vi "Color detect test.vi"(0 "Image 3":T2(plugin-control)) -> (1 "Image":T2(plugin-control), 2 "Enum":enum16{"Z", "I", "O", "S", "L", "J", "T", "N"}(ring))   [LabVIEW 2015]
uses:
  <vilib>/vision/Image Controls.llb/IMAQ Image.ctl
  <vilib>/vision/NI_Vision_Development_Module.lvlib
panel:
  in  "output cluster 2":T1(array[cluster])
  out "Area":dbl[](array[numeric])
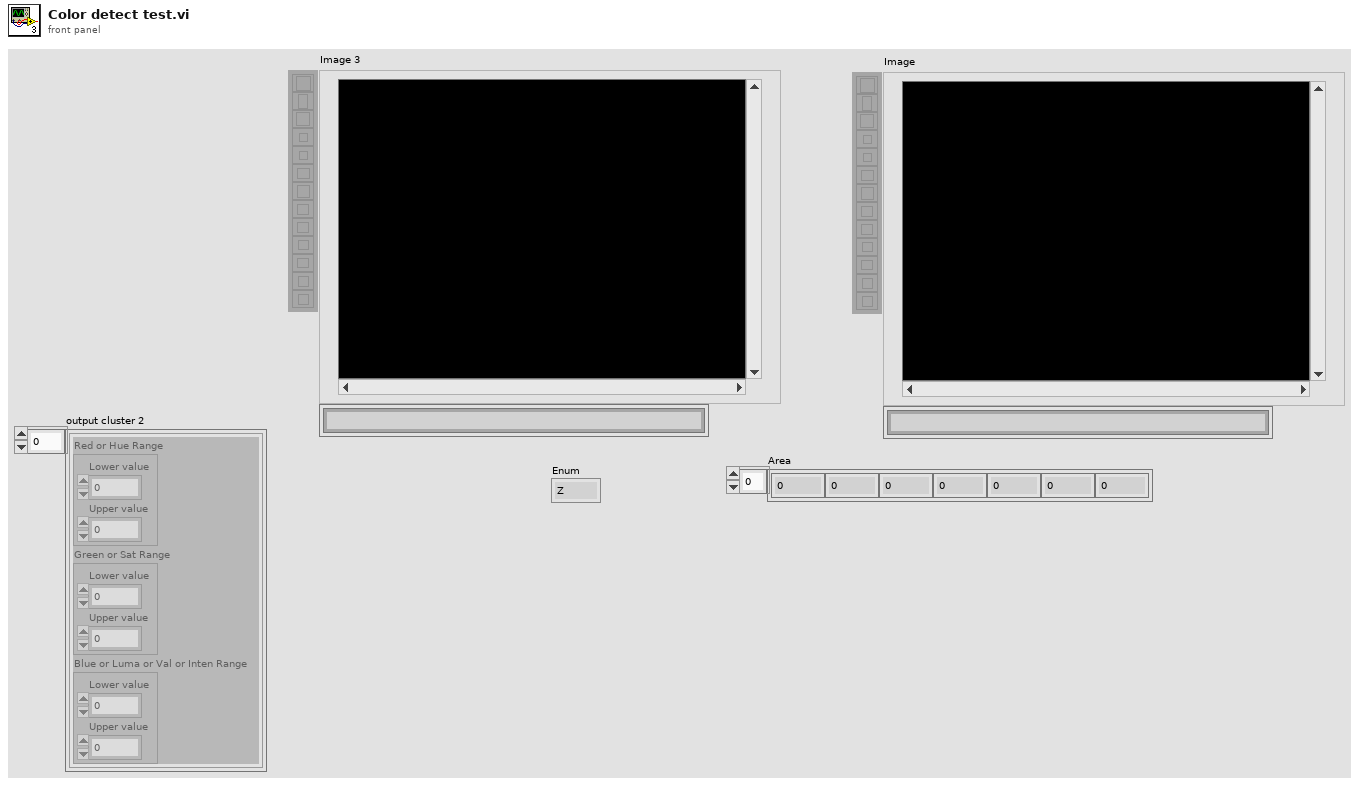
[diagram p1: front panel]
types:
  T1 = cluster{"Red or Hue Range":cluster{"Lower value":i32, "Upper value":i32}, "Green or Sat Range":cluster{"Lower value":i32, "Upper value":i32}, "Blue or Luma or Val or Inten Range":cluster{"Lower value":i32, "Upper value":i32}}[]
  T2 = typedef "IMAQ Image.ctl" = refnum<image>
  T3 = typedef "Particle Parameters" = i32
  T4 = cluster{"Red or Hue Range":cluster{"Lower value":i32, "Upper value":i32}, "Green or Sat Range":cluster{"Lower value":i32, "Upper value":i32}, "Blue or Luma or Val or Inten Range":cluster{"Lower value":i32, "Upper value":i32}}
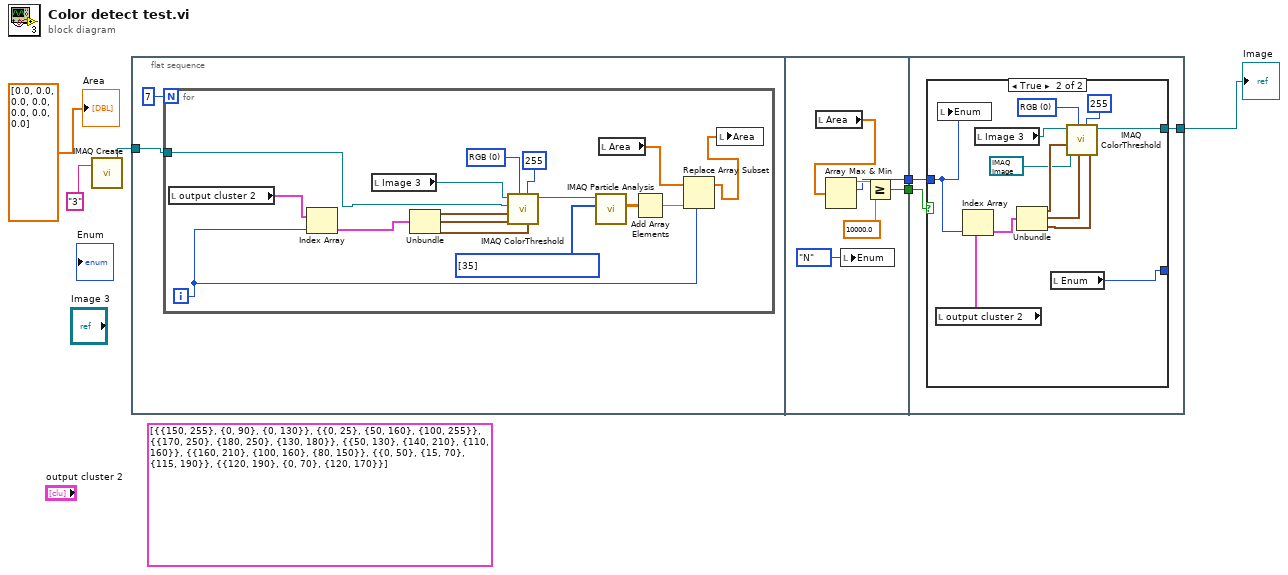
[diagram p0: block diagram]
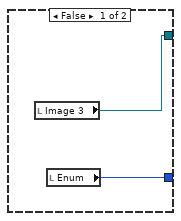
[diagram p2: hidden frame]
diagram:
  (unwired) T1 [{"Red or Hue Range"={"Lower value"=150, "Upper value"=255}, "Green or Sat Range"={"Lower value"=0, "Upper value"=90}, "Blue or Luma or Val or Inten Range"={"Lower value"=0, "Upper value"=130}}, {"Red or Hue Range"={"Lower value"=0, "Upper value"=25}, "Green or Sat Range"={"Lower value"=50, "Upper value"=160}, "Blue or Luma or Val or Inten Range"={"Lower value"=100, "Upper value"=255}}, {"Red or Hue Range"={"Lower value"=170, "Upper value"=250}, "Green or Sat Range"={"Lower value"=180, "Upper value"=250}, "Blue or Luma or Val or Inten Range"={"Lower value"=130, "Upper value"=180}}, {"Red or Hue Range"={"Lower value"=50, "Upper value"=130}, "Green or Sat Range"={"Lower value"=140, "Upper value"=210}, "Blue or Luma or Val or Inten Range"={"Lower value"=110, "Upper value"=160}}, {"Red or Hue Range"={"Lower value"=160, "Upper value"=210}, "Green or Sat Range"={"Lower value"=100, "Upper value"=160}, "Blue or Luma or Val or Inten Range"={"Lower value"=80, "Upper value"=150}}, {"Red or Hue Range"={"Lower value"=0, "Upper value"=50}, "Green or Sat Range"={"Lower value"=15, "Upper value"=70}, "Blue or Luma or Val or Inten Range"={"Lower value"=115, "Upper value"=190}}, {"Red or Hue Range"={"Lower value"=120, "Upper value"=190}, "Green or Sat Range"={"Lower value"=0, "Upper value"=70}, "Blue or Luma or Val or Inten Range"={"Lower value"=120, "Upper value"=170}}] ("output cluster 3")
  n1 = call "IMAQ Create"("Image Name"="3") -> ("New Image"=w1:T2)  [unwired: 4 in, 1 out]
  n2 = flat-sequence {
    tunnel: w1 -> [w7]
    tunnel: [w27] -> w6
    tunnel: [w26] -> w5
    tunnel: w6 -> [w33]
    tunnel: w5 -> [w32]
    tunnel: [w31] -> w4
    frame #0 {
      n3 = for {
        N: 7 -> [_]
        tunnel: w7 -> [w10]
        i -> [w13]
        w23 = T3[] [35] items=["Center of Mass X", "Center of Mass Y", "First Pixel X", "First Pixel Y", "Bounding Rect Left", "Bounding Rect Top", "Bounding Rect Right", "Bounding Rect Bottom", "Max Feret Diameter Start X", "Max Feret Diameter Start Y", "Max Feret Diameter End X", "Max Feret Diameter End Y", "Max Horiz. Segment Length Left", "Max Horiz. Segment Length Right", "Max Horiz. Segment Length Row", "-", "Bounding Rect Width", "Bounding Rect Height", "Bounding Rect Diagonal", "Perimeter", "Convex Hull Perimeter", "Holes' Perimeter", "Max Feret Diameter", "Equivalent Ellipse Major Axis", "Equivalent Ellipse Minor Axis", "Equivalent Ellipse Minor Axis (Feret)", "Equivalent Rect Long Side", "Equivalent Rect Short Side", "Equivalent Rect Diagonal", "Equivalent Rect Short Side (Feret)", "Average Horiz. Segment Length", "Average Vert. Segment Length", "Hydraulic Radius", "Waddel Disk Diameter", "-", "Area", "Holes' Area", "Particle & Holes' Area", "Convex Hull Area", "Image Area", "-", "Number of Holes", "Number of Horiz. Segments", "Number of Vert. Segments", "-", "Orientation", "Max Feret Diameter Orientation", "-", "% Area/Image Area", "% Area/(Particle & Holes' Area)", "Ratio of Equivalent Ellipse Axes", "Ratio of Equivalent Rect Sides", "-", "Elongation Factor", "Compactness Factor", "Heywood Circularity Factor", "Type Factor", "-", "Sum X", "Sum Y", "Sum XX", "Sum XY", "Sum YY", "Sum XXX", "Sum XXY", "Sum XYY", "Sum YYY", "-", "Moment of Inertia XX", "Moment of Inertia XY", "Moment of Inertia YY", "Moment of Inertia XXX", "Moment of Inertia XXY", "Moment of Inertia XYY", "Moment of Inertia YYY", "Norm. Moment of Inertia XX", "Norm. Moment of Inertia XY", "Norm. Moment of Inertia YY", "Norm. Moment of Inertia XXX", "Norm. Moment of Inertia XXY", "Norm. Moment of Inertia XYY", "Norm. Moment of Inertia YYY", "Hu Moment 1", "Hu Moment 2", "Hu Moment 3", "Hu Moment 4", "Hu Moment 5", "Hu Moment 6", "Hu Moment 7"] ("Pixel Measurements")
        w24 = u16 0 items=["RGB", "HSL", "HSV", "HSI"] ("Color Mode")
        n4 = local read "output cluster 2"() -> (w14:T1)
        n5 = Index Array(array=w14, index=w13) -> (element=w16:T4)
        n6 = local read "Image 3"() -> (w9:T2)
        n7 = Unbundle(w16) -> ("Red or Hue Range"=w21:cluster{"Lower value":i32, "Upper value":i32}, "Green or Sat Range"=w20:cluster{"Lower value":i32, "Upper value":i32}, "Blue or Luma or Val or Inten Range"=w17:cluster{"Lower value":i32, "Upper value":i32})
        n8 = call "IMAQ ColorThreshold"("Blue or Luma or Val or Inten Range"=w17, "Replace Value"=255, "Green or Sat Range"=w20, "Color Mode"=w24, "Red or Hue Range"=w21, "Image Dst"=w10, "Image Src"=w9) -> ("Image Dst Out"=w18:T2)  [unwired: 3 in, 1 out]
        n9 = call "IMAQ Particle Analysis"("Pixel Measurements"=w23, "Image"=w18) -> ("Particle Measurements (Pixels)"=w22:dbl[][])  [unwired: 4 in, 5 out]
        n10 = local read "Area"() -> (w12:dbl[])
        n11 = Add Array Elements(numeric array=w22) -> (sum=w15:dbl)
        n12 = Replace Array Subset(array=w12, new element=w15, index=w13) -> (w11:dbl[])
        n13 = local write "Area"(w11) -> ()
      }
    }
    frame #1 {
      n14 = local read "Area"() -> (w30:dbl[])
      n15 = Array Max & Min(array=w30) -> (max value=w29:dbl, max index (indices)=w26:i32)  [unwired: 2 out]
      n16 = local write "Enum"(enum16{"Z", "I", "O", "S", "L", "J", "T", "N"}."N" ("Enum")) -> ()
      n17 = Greater Or Equal?(x=w29, y=10000.0) -> (x >= y?=w27:bool)
    }
    frame #2 {
      n18 = case shown="True" w33 {
        tunnel: w32 -> [_ w43]
        tunnel: [w35 w44] -> w31
        tunnel: [w34 w36] -> _
        frame False {
          n19 = local read "Image 3"() -> (w35:T2)
          n20 = local read "Enum"() -> (w34:enum16{"Z", "I", "O", "S", "L", "J", "T", "N"})
        }
        frame True {
          w46 = u16 0 items=["RGB", "HSL", "HSV", "HSI"] ("Color Mode")
          n21 = local read "output cluster 2"() -> (w42:T1)
          n22 = local write "Enum"(w43) -> ()
          n23 = Index Array(array=w42, index=w43) -> (element=w41:T4)
          n24 = local read "Image 3"() -> (w47:T2)
          n25 = Unbundle(w41) -> ("Red or Hue Range"=w40:cluster{"Lower value":i32, "Upper value":i32}, "Green or Sat Range"=w39:cluster{"Lower value":i32, "Upper value":i32}, "Blue or Luma or Val or Inten Range"=w38:cluster{"Lower value":i32, "Upper value":i32})
          n26 = local read "Enum"() -> (w36:enum16{"Z", "I", "O", "S", "L", "J", "T", "N"})
          n27 = call "IMAQ ColorThreshold"("Blue or Luma or Val or Inten Range"=w38, "Replace Value"=255, "Green or Sat Range"=w39, "Color Mode"=w46, "Red or Hue Range"=w40, "Image Dst"=T2 refnum, "Image Src"=w47) -> ("Image Dst Out"=w44:T2)  [unwired: 3 in, 1 out]
        }
      }
    }
  }
  "Image" <- w4
  "Area" <- dbl[] [0.0, 0.0, 0.0, 0.0, 0.0, 0.0, 0.0] ("Area")
